vi "DLT.vi"(0 "System no.":i32=1 min=1 max=4 step=1, 2 "File Name":string, 5 "error in":errorcluster) -> (19 "error out":errorcluster)   [LabVIEW 2026]
doc: "Deletes a data file that was saved in nonvolatile memory using the STD command.\nDeleting a data file with DLT requires switching to command level 1 with the CCL command\n\nE-754: Check HLP? answer to find out if DLT is supported"
panel:
  # "Deletes a data file that was saved in non-volatile memory using the STD command."
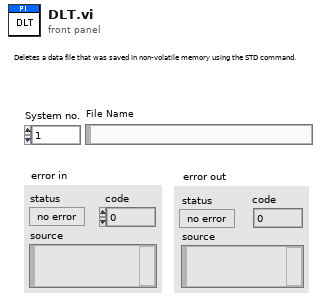
[diagram p1: front panel]
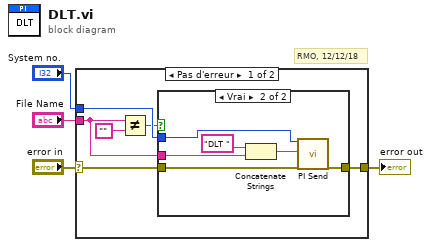
[diagram p0: block diagram]
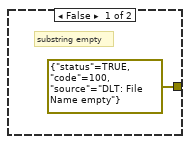
[diagram p2: hidden frame]
diagram:
  # "RMO, 12/12/18"
  n1 = case shown="Pas d'erreur" "error in" {
    selector: "error in" -> [w9 w18]
    tunnel: [w10 w18] -> w4
    tunnel: "System no." -> [w8 _]
    tunnel: "File Name" -> [w5 _]
    frame No Error {
      n2 = Not Equal?(x=w5, y="") -> (x != y?=w6:bool)
      n3 = case shown="Vrai" w6 {
        tunnel: [errorcluster {"status"=TRUE, "code"=100, "source"="DLT: File Name empty"} ("error out") w16] -> w10
        tunnel: w9 -> [_ w17]
        tunnel: w8 -> [_ w15]
        tunnel: w5 -> [_ w13]
        frame False {
          # "substring empty"
        }
        frame True {
          n4 = Concatenate Strings("DLT ", w13) -> (w12:string)
          n5 = call "PI Send.vi"("System no."=w15, "String to send"=w12, "error in"=w17) -> ("error out"=w16:errorcluster)  [unwired: 3 in, 13 out]
        }
      }
    }
    frame Error {
    }
  }
  "error out" <- w4
